vi "Clean.vi"(0 "Installer_LV in":refnum<class "Installer_LV.lvclass">) -> (4 "Installer_LV out":refnum<class "Installer_LV.lvclass">)   [LabVIEW 2017, in "CL_G3_VIComponentBuilder.lvlib" / "Installer_LV.lvclass"]
doc: "Deletes the directory in which the installer is located from the Component's Export directory. The installer is located in a directory named after the installer's build spec name."
uses:
  Installer_LV.lvclass
  C:/builds/Component BuilderBT/SrcDist/Exports/Exports/Export.lvclass
  C:/builds/Component BuilderBT/SrcDist/Exports/NI Build Specification_LV/NI Build Specification_LV.lvclass
  Exports/Export.lvclass/Export.ctl
  NI Build Specification_LV/NI Build Specification_LV.lvclass/NI Build Specification_LV.ctl
  Exports/Accessors/Read Component Export Dir.vi
  NI Build Specification_LV/Accessors/Read Export's Build Spec Name.vi
  NI Build Specification_LV/NI Build Specification_LV.lvclass
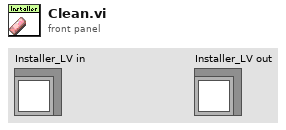
[diagram p1: front panel]
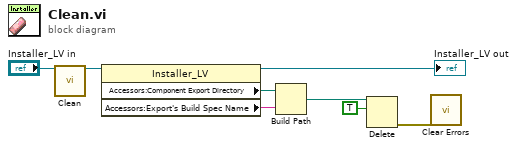
[diagram p0: block diagram]
diagram:
  n1 = call-parent "Clean.vi"("NI Build Specification_LV in"="Installer_LV in") -> ("NI Build Specification_LV out"=w7:refnum<class "Installer_LV.lvclass">)  [unwired: 14 in]
  n2 = property class="Installer_LV"(reference=w7) -> (reference out=→"Installer_LV out":refnum<class "Installer_LV.lvclass">, "Accessors:Component Export Directory"=w5:path, "Accessors:Export's Build Spec Name"=w4:string)  [unwired: 1 in, 1 out]
  n3 = Build Path(base path=w5, name or relative path=w4) -> (appended path=w3:path)
  n4 = Delete(path (use dialog)=w3, entire hierarchy (F)=TRUE) -> (error out=w1:errorcluster)  [unwired: 3 in, 2 out]
  n5 = call <vilib>:"Clear Errors.vi"("error in (no error)"=w1) -> ()  [unwired: 5 in, 2 out]
